vi "fluoroprobe DECODE.vi"(11 "input string":string) -> (0 "检测浓度":T1, 1 "555 string":string, 2 "553 string":string, 3 "output string":string)   [LabVIEW 2016, in "bbe.lvlib"]
uses:
  <vilib>/regexp/Match Regular Expression.xnode
  bbe.lvlib
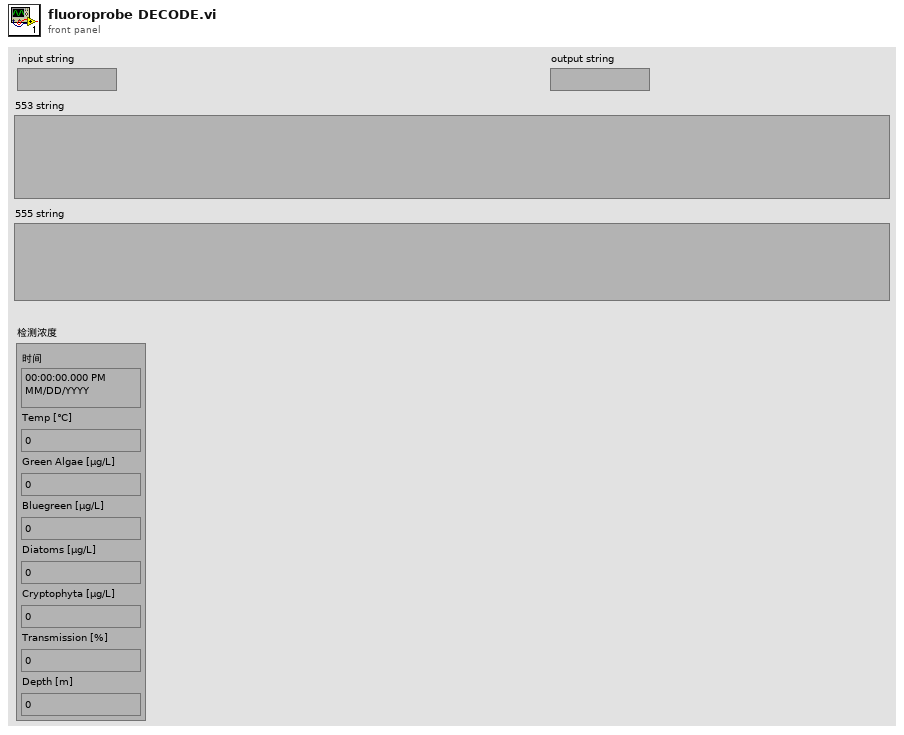
[diagram p1: front panel]
types:
  T1 = cluster{"时间":timestamp, "Temp [℃]":dbl, "Green Algae [μg/L]":dbl, "Bluegreen [μg/L]":dbl, "Diatoms [μg/L]":dbl, "Cryptophyta [μg/L]":dbl, "Transmission [%]":dbl, "Depth [m]":dbl}
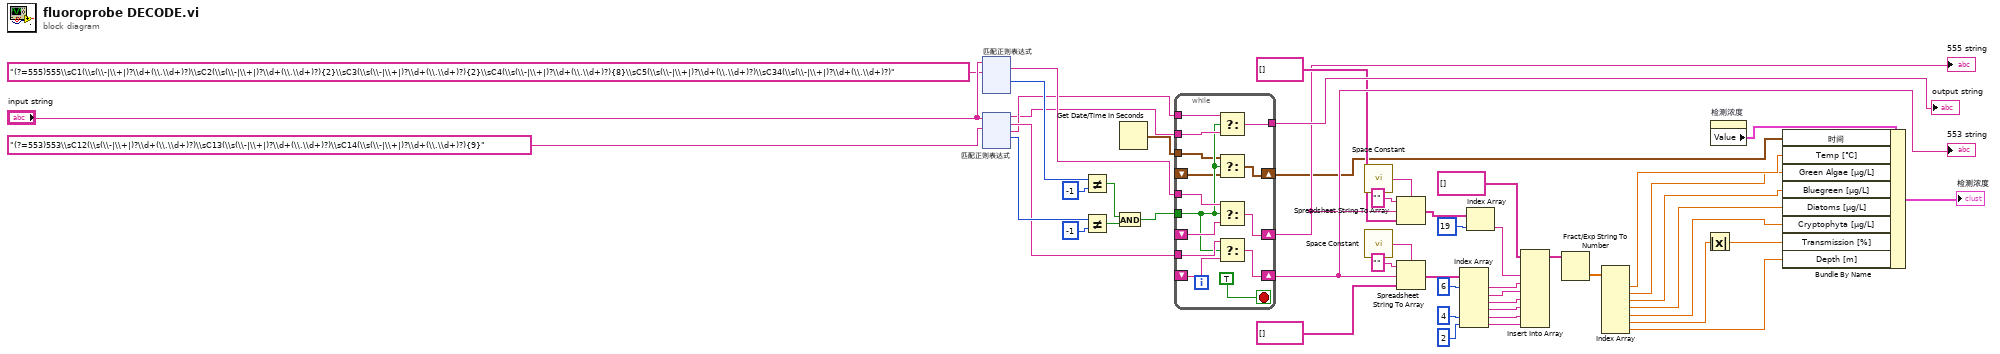
[diagram p0: block diagram]
diagram:
  n1 = xnode "匹配正则表达式"("输入字符串"="input string", "正则表达式"="(?=555)555\\sC1(\\s(\\-|\\+|)?\\d+(\\.\\d+)?)\\sC2(\\s(\\-|\\+|)?\\d+(\\.\\d+)?){2}\\sC3(\\s(\\-|\\+|)?\\d+(\\.\\d+)?){2}\\sC4(\\s(\\-|\\+|)?\\d+(\\.\\d+)?){8}\\sC5(\\s(\\-|\\+|)?\\d+(\\.\\d+)?)\\sC34(\\s(\\-|\\+|)?\\d+(\\.\\d+)?)") -> ("所有匹配"=w42:string, "匹配后偏移量"=w46:i32)  [unwired: 4 in, 3 out]
  n2 = xnode "匹配正则表达式"("输入字符串"="input string", "正则表达式"="(?=553)553\\sC12(\\s(\\-|\\+|)?\\d+(\\.\\d+)?)\\sC13(\\s(\\-|\\+|)?\\d+(\\.\\d+)?)\\sC14(\\s(\\-|\\+|)?\\d+(\\.\\d+)?){9}") -> ("匹配之前"=w38:string, "所有匹配"=w41:string, "匹配之后"=w39:string, "匹配后偏移量"=w48:i32)  [unwired: 4 in, 1 out]
  n3 = Not Equal?(x=w46, y=-1) -> (x != y?=w50:bool)
  n4 = Not Equal?(x=w48, y=-1 ("匹配后偏移量")) -> (x != y?=w49:bool)
  n5 = And(x=w50, y=w49) -> (x .and. y?=w40:bool)
  n6 = Get Date/Time In Seconds() -> (seconds since 1Jan1904=w3:timestamp)
  n7 = while {
    shift-right: [w63] -> w29
    shift-left: _ -> [w62]
    tunnel: w42 -> [w64]
    shift-right: [w60] -> w35
    shift-left: _ -> [w59]
    tunnel: w41 -> [w61]
    tunnel: w40 -> [w55]
    tunnel: w39 -> [w58]
    tunnel: w38 -> [w57]
    tunnel: [w56] -> w33
    shift-right: [w53] -> w2
    shift-left: _ -> [w52]
    tunnel: w3 -> [w54]
    stop <- TRUE stop-if-true
    n8 = Select(t=w58, s=w55, f=w57) -> (s? t:f=w56:string)
    n9 = Select(t=w54, s=w55, f=w52) -> (s? t:f=w53:timestamp)
    n10 = Select(t=w64, s=w55, f=w62) -> (s? t:f=w63:string)
    n11 = Select(t=w61, s=w55, f=w59) -> (s? t:f=w60:string)
  }
  "output string" <- w33
  "555 string" <- w29
  "553 string" <- w35
  n12 = call <vilib>:"Space Constant.vi"() -> ("String"=w30:string)
  n13 = call <vilib>:"Space Constant.vi"() -> ("String"=w34:string)
  n14 = Spreadsheet String To Array(delimiter (Tab)=w30, format string="" ("格式字符串"), spreadsheet string=w29, array type (2D Dbl)=string[] []) -> (array=w28:string[])
  n15 = Spreadsheet String To Array(delimiter (Tab)=w34, format string="" ("电子表格字符串"), spreadsheet string=w35, array type (2D Dbl)=string[] []) -> (array=w26:string[])
  n16 = Index Array(array=w26, index #1=6 ("索引"), index #5=4 ("索引"), index #6=2 ("索引")) -> (element #1=w21:string, element #2=w20:string, element #3=w19:string, element #4=w18:string, element #5=w17:string, element #6=w16:string)  [unwired: 3 in]
  n17 = Index Array(array=w28, index=19 ("索引")) -> (element=w22:string)
  n18 = Insert Into Array(array=string[] [] ("数组"), new element #1=w22, new element #2=w21, new element #3=w20, new element #4=w19, new element #5=w18, new element #6=w17, new element #7=w16) -> (w14:string[])  [unwired: 1 in]
  n19 = Fract/Exp String To Number(string=w14) -> (number=w11:dbl[])  [unwired: 3 in, 1 out]
  n20 = Index Array(array=w11) -> (element #1=w10:dbl, element #2=w9:dbl, element #3=w8:dbl, element #4=w7:dbl, element #5=w6:dbl, element #6=w5:dbl, element #7=w4:dbl)  [unwired: 7 in]
  n21 = Absolute Value(x=w5) -> (abs(x)=w1:dbl)
  n22 = property on="检测浓度" class="Clust (严格)"() -> ("Value"=w13:T1)  [unwired: 2 in, 2 out]
  n23 = Bundle By Name(cluster=w13, "时间"=w2, "Temp [℃]"=w10, "Green Algae [μg/L]"=w9, "Bluegreen [μg/L]"=w8, "Diatoms [μg/L]"=w7, "Cryptophyta [μg/L]"=w6, "Transmission [%]"=w1, "Depth [m]"=w4) -> (→"检测浓度":T1)
